vi "Wait.Gui.Kill.vi"(8 "error in (no error)":errorcluster) -> (0 "error out":errorcluster)   [LabVIEW 2016]
uses:
  Wait.Gui.Action.ctl
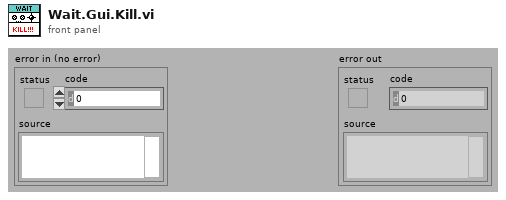
[diagram p1: front panel]
types:
  T1 = typedef "Wait.Gui.Action.ctl" = enum32{"idle", "constructor", "destructor", "--- WaitGui ---", "open FP", "close FP", "update msg", "update progbar"}
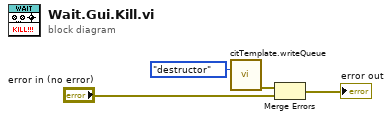
[diagram p0: block diagram]
diagram:
  n1 = call "citTemplate.writeQueue.vi"("event in (if not connected:all statemachine with data event)"=Wait.Gui.Action."destructor" ("Action")) -> ("error out"=w1:errorcluster)  [unwired: 14 in]
  n2 = Merge Errors(w1, "error in (no error)") -> (→"error out":errorcluster)
